vi "Auto Fire.vi"(10 "Robot Commands 2":T1, 11 "Robot Commands":T1) -> ()   [LabVIEW 2014]
uses:
  SubSystems/Robot Commands.ctl
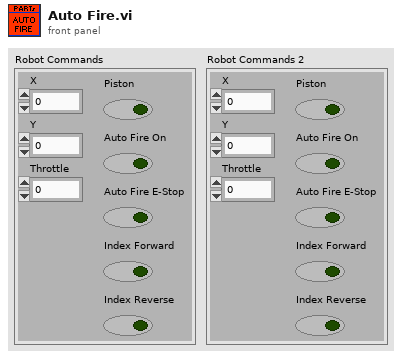
[diagram p1: front panel]
types:
  T1 = typedef "Robot Commands.ctl" = cluster{"X":dbl, "Y ":dbl, "Throttle":dbl, "Piston":bool, "Auto Fire On":bool, "Auto Fire E-Stop":bool, "Index Forward":bool, "Index Reverse ":bool}
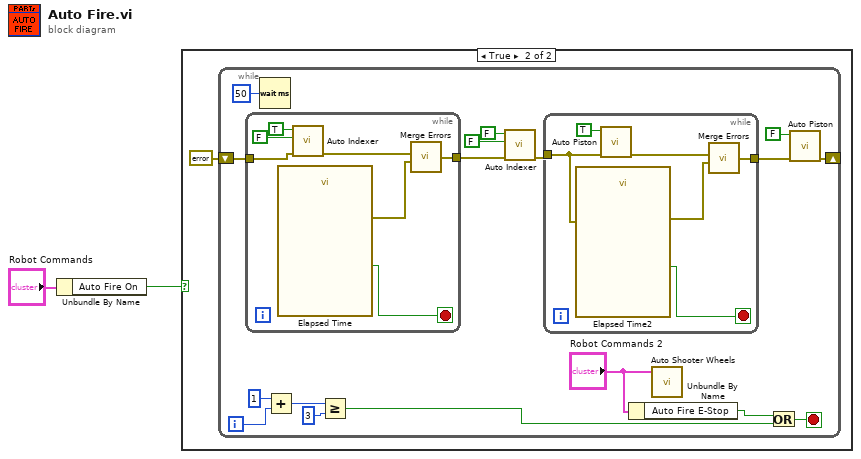
[diagram p0: block diagram]
diagram:
  n1 = Unbundle By Name("Robot Commands") -> ("Auto Fire On"=w1:bool)
  n2 = case shown="True" w1 {
    frame False {
    }
    frame True {
      n3 = while {
        shift-right: [w5] -> _
        shift-left: errorcluster {"status"=FALSE, "code"=0, "source"=""} ("error out") -> [w4]
        i -> [w12]
        stop <- w8 stop-if-true
        n4 = while {
          tunnel: [w28] -> w18
          tunnel: w4 -> [w27]
          stop <- w31 stop-if-true
          n5 = call "Elapsed Time"() -> ("Time has Elapsed"=w31:bool, "error out"=w29:errorcluster)  [unwired: 12 in, 6 out]
          n6 = call "Auto Indexer.vi"("error in (no error)"=w27, "T=Reverse"=FALSE ("F=Reverse"), "T=Forward"=TRUE) -> ("error out"=w30:errorcluster)  [unwired: 8 in]
          n7 = call "Merge Errors.vi"("error in 2"=w29, "error in"=w30) -> ("error out"=w28:errorcluster)  [unwired: 2 in]
        }
        n8 = Wait (ms)(milliseconds to wait=u32 50) -> ()  [unwired: 1 out]
        n9 = Add(x=1, y=w12) -> (x+y=w10:i32)
        n10 = Greater Or Equal?(x=w10, y=3) -> (x >= y?=w6:bool)
        n11 = call "Auto Indexer.vi"("error in (no error)"=w18, "T=Reverse"=FALSE ("F=Reverse"), "T=Forward"=FALSE) -> ("error out"=w17:errorcluster)  [unwired: 8 in]
        n12 = while {
          tunnel: [w24] -> w15
          tunnel: w17 -> [w21]
          stop <- w26 stop-if-true
          n13 = call "Elapsed Time2"("error in (no error)"=w21) -> ("Time has Elapsed"=w26:bool, "error out"=w25:errorcluster)  [unwired: 11 in, 6 out]
          n14 = call "Auto Piston.vi"("error in (no error)"=w21, "T=Forward, F=Reverse"=TRUE) -> ("error out"=w23:errorcluster)  [unwired: 9 in]
          n15 = call "Merge Errors.vi"("error in 2"=w25, "error in"=w23) -> ("error out"=w24:errorcluster)  [unwired: 2 in]
        }
        n16 = Unbundle By Name("Robot Commands 2") -> ("Auto Fire E-Stop"=w7:bool)
        n17 = call "Auto Shooter Wheels.vi"("Robot Commands"="Robot Commands 2") -> ()  [unwired: 10 in, 1 out]
        n18 = Or(x=w7, y=w6) -> (x .or. y?=w8:bool)
        n19 = call "Auto Piston.vi"("error in (no error)"=w15, "T=Forward, F=Reverse"=FALSE) -> ("error out"=w5:errorcluster)  [unwired: 9 in]
      }
    }
  }
